vi "GlueRepeatedLinePattern.vi"(2 "Controller In":refnum<k24>, 3 "Dry Run":bool, 4 "Stereo Angle [mrad]":dbl=-26.0 format="%#_13g", 5 "Module Number":i32=7, 6 "Calibration Directory":path) -> (0 ".NET Refnum out":refnum<k24>)   [LabVIEW 2016]
uses:
  <vilib>/LabVIEW Interface for Arduino/Type Defs/Arduino Resource.ctl
  <vilib>/LabVIEW Interface for Arduino/Type Defs/Board Type.ctl
  C:/Users/Aerotech/Documents/BNLStaveAssembly-blueprint/Bin/Aerotech.A3200.dll
  BNLStaveAssembly-blueprint/Bin/Aerotech.A3200.dll
  <vilib>/LabVIEW Interface for Arduino/Type Defs/Pin Mode.ctl
  <vilib>/Utility/file.llb/Read Delimited Spreadsheet (DBL).vi
  <vilib>/LabVIEW Interface for Arduino/LabVIEW Interface for Arduino.lvlib
panel:
  out "Shift to Start [mm]":dbl[](array[numeric])
  out "Calibrated Start [mm]":dbl[](array[numeric])
  out "Start Position [mm]":dbl[](array[numeric])
  out "Line Motion":T1
  out "N Lines":i32
  out "Lines Glued":i32
  out "Elapsed Time [s]":dbl format="%.2g"
  out "Finished":bool
  in  "Abort stage":bool
  in  "Pattern Indicator":enum32{"Glue Pattern"}(tab)
  out "Relative Line\nSeparations [mm]":dbl[][](array[numeric])=[[18.5, 7.25], [2.5, 3.5], [-3.5, 5.0], [2.5, 3.15], [2.5, 3.15], [2.5, 3.15], [2.5, 3.15], [2.5, 3.15], [2.5, 3.15], [2.5, 3.15], [2.5, 3.15], [2.5, 3.15], [2.5, 3.15], [2.5, 3.15], [3.75, 5.0], [2.5, 3.5]] format="%#_13g"
  out "Line Lengths [mm]":dbl[](array[numeric])=[65.0, 65.0, 73.5, 73.5, 73.5, 73.5, 73.5, 73.5, 73.5, 73.5, 73.5, 73.5, 73.5, 73.5, 65.0, 65.0] format="%#_13g"
  in  "Outputs Tab":enum32{"Running Positions"}(tab)
  out "Running Positions [mm]":dbl[][](array[numeric])
  in  "Times [s]":dbl[](array[numeric])
  out "Running Times [s]":dbl[](array[numeric])
  in  "Inputs Tab":T2(tab)
  out "Virtual Stave Map":path
  out "Stave Angle [rad]":dbl format="%#_13g"
  out "Total Angle [rad]":dbl
  out "Orientation":string
  out "Pin Down?":bool
  in  "Pulse Length [ms]":dbl=125.0 format="%#_13g"
  out "Arduino Resource":T3={"VISA resource"="GlueCTRL", "Board Type"=enum."Uno", "Connection Type"=enum."USB / Serial", "Bytes Per Packet (15)"=15}
  in  "Digital I/O Pin":u8=7
  in  "Default Axis Speeds":T5={"X [mm/s]"=25.0, "Y [mm/s]"=25.0, "Z [mm/s]"=25.0}
  in  "Camera to Dispenser \nShift [mm]":dbl[](array[numeric])=[109.832, 5.121, 0.0]
  in  "Glue Pattern .csv File":path=path "C:/Users/Aerotech/Documents/BNL_ThermomechanicalStave/Glue/GluePatterns/Pattern6-0.txt"
  in  "Axial":bool=TRUE
  in  "Motion Time per Line [s]":dbl=4.35 format="%#_13g"
  in  "Wait [ms]":dbl=750.0 format="%#_13g"
  in  "Positions [mm]":dbl[][](array[numeric])
  in  "Terminate":bool
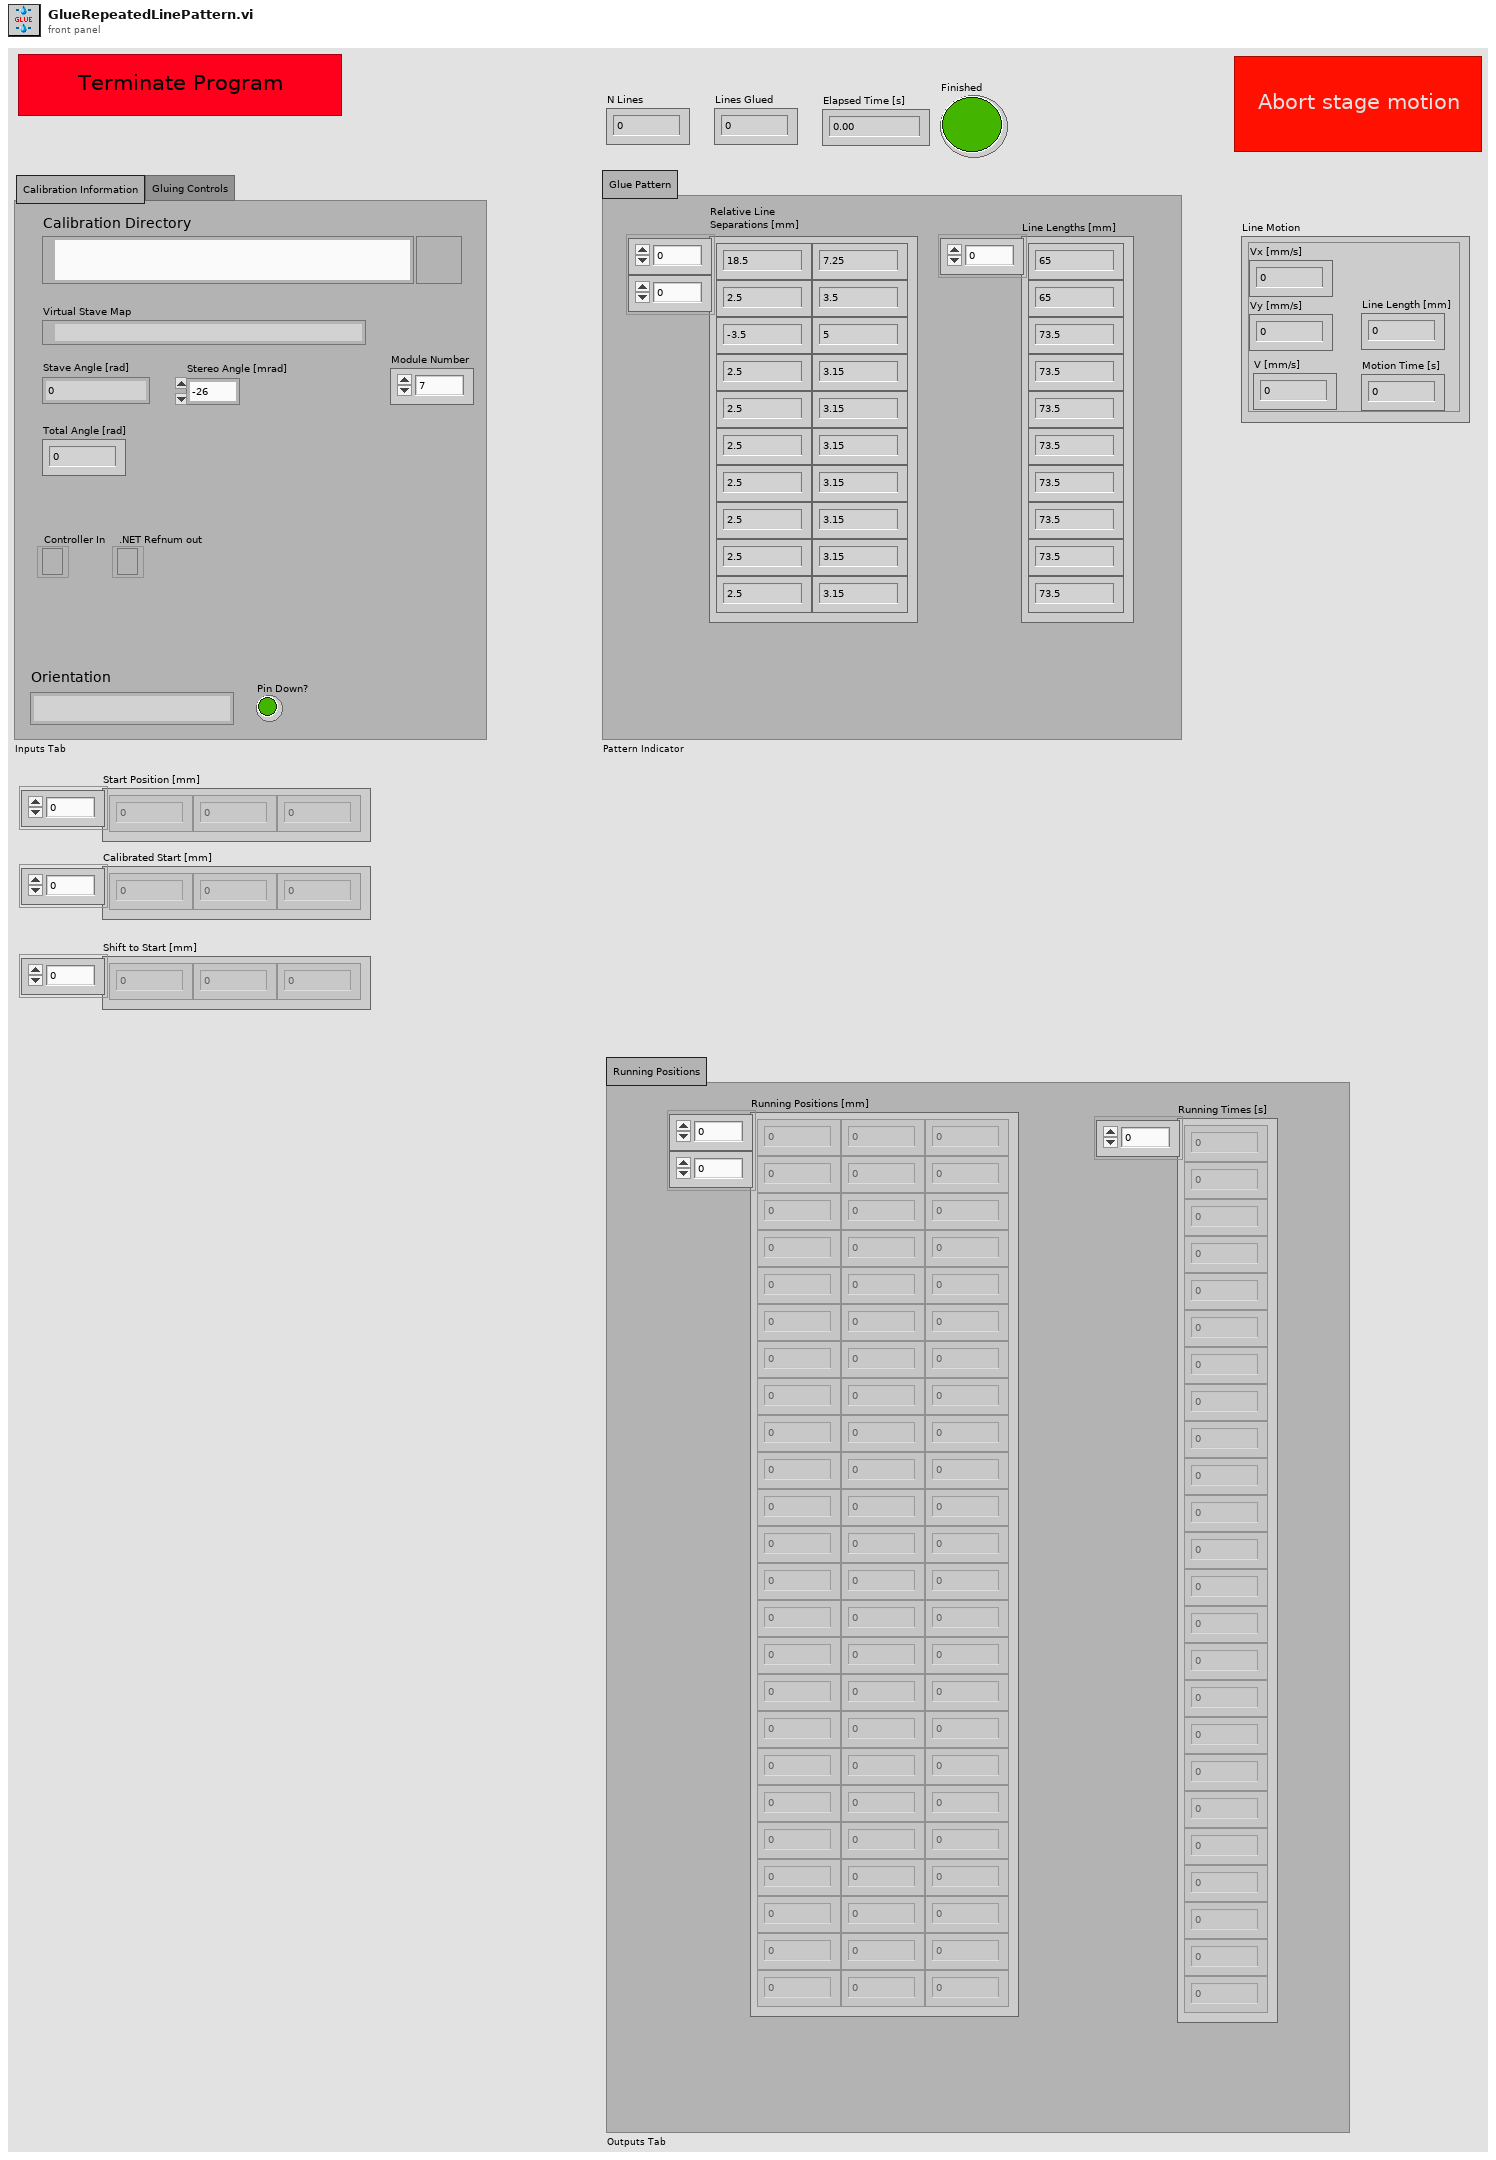
[diagram p1: front panel]
types:
  T1 = cluster{"Vx [mm/s]":dbl, "Vy [mm/s]":dbl, "Numeric Control":dbl, "Numeric Control":dbl, "Line Length [mm]":dbl}
  T2 = enum32{"Calibration Information", "Gluing Controls"}
  T3 = typedef "LabVIEW Interface for Arduino.lvlib/Arduino Resource.ctl" = cluster{"VISA resource":refnum<visa-resource-name>, "Board Type":T4, "Connection Type":enum8{"USB / Serial"}, "Bytes Per Packet (15)":u8}
  T4 = typedef "LabVIEW Interface for Arduino.lvlib/Board Type.ctl" = enum16{"Uno", "Dimuelanove w/Atmega 328", "Mega 2560"}
  T5 = cluster{"X [mm/s]":dbl, "Y [mm/s]":dbl, "Z [mm/s]":dbl}
  T6 = typedef "LabVIEW Interface for Arduino.lvlib/Pin Mode.ctl" = enum8{"Input", "Output"}
  T7 = cluster{"X [mm]":dbl, "Y [mm]":dbl, "Z [mm]":dbl}
  T8 = cluster{"Final X":dbl, "Final Y":dbl, "Final Z":dbl}
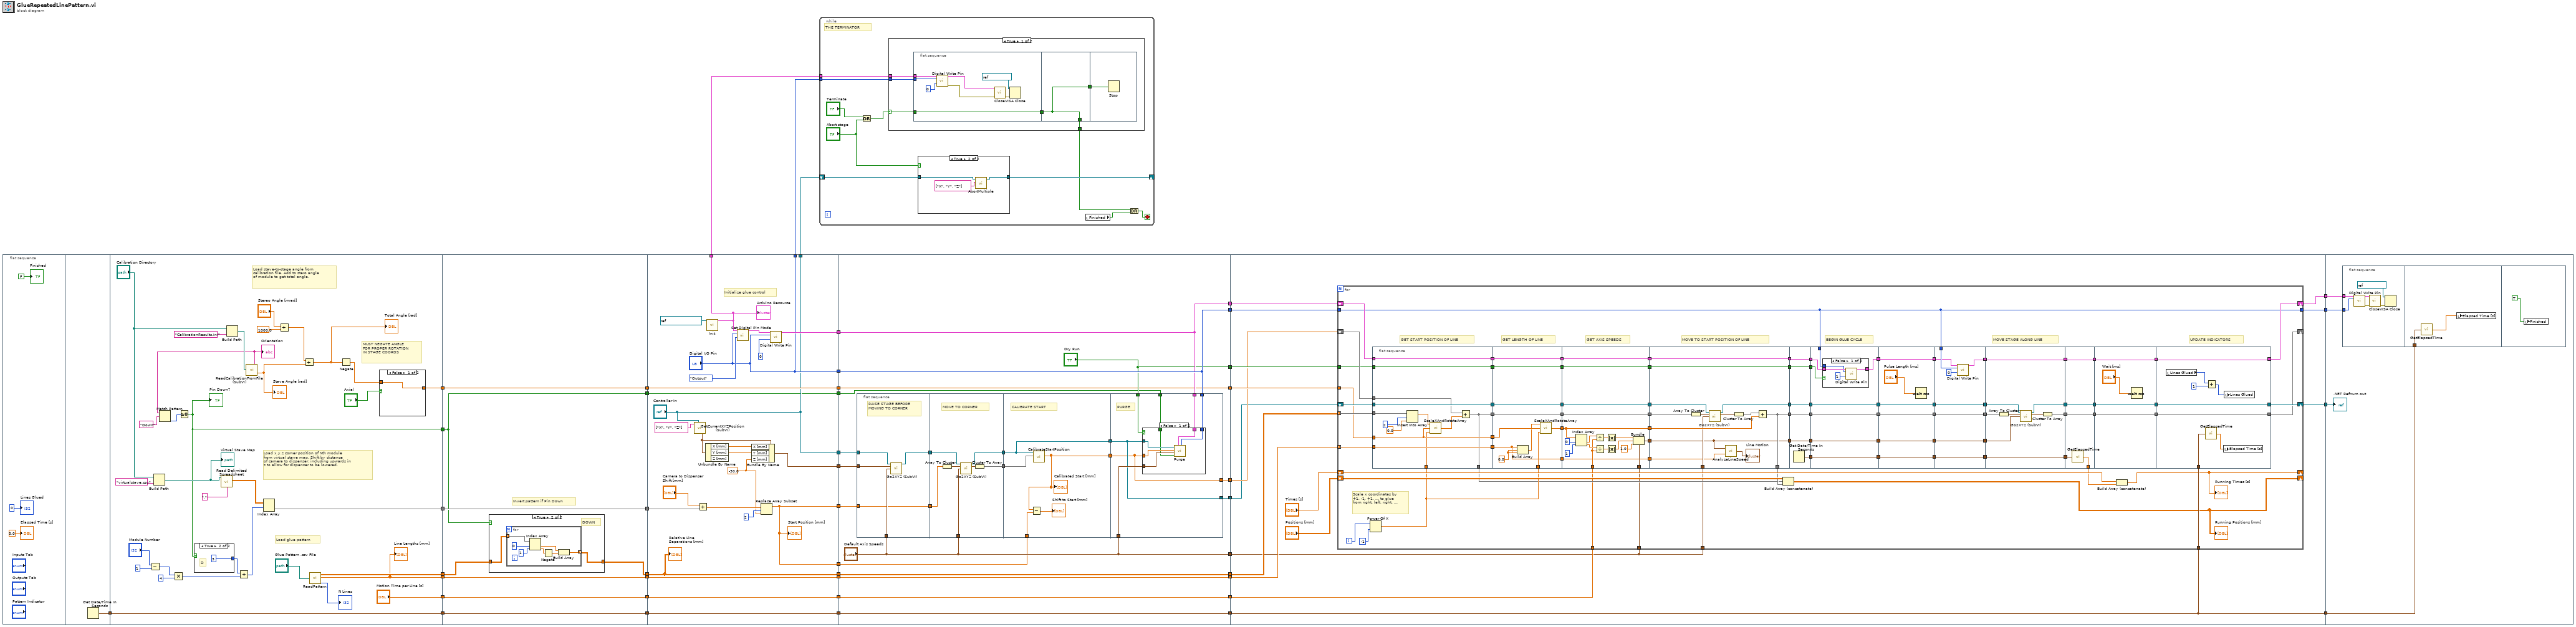
[diagram p0: block diagram]
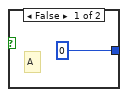
[diagram p2: hidden frame]
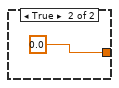
[diagram p3: hidden frame]
diagram:
  n1 = flat-sequence {
    tunnel: [w49] -> w31
    tunnel: w31 -> [w69]
    tunnel: [w69] -> w16
    tunnel: [w63] -> w14
    tunnel: [w66] -> w12
    tunnel: [w65] -> w10
    tunnel: [w62] -> w8
    tunnel: ["Motion Time per Line [s]"] -> w6
    tunnel: [w50] -> w4
    tunnel: w16 -> [w94]
    tunnel: [w94] -> w15
    tunnel: w14 -> [w93]
    tunnel: [w93] -> w13
    tunnel: w12 -> [w89]
    tunnel: [w88] -> w11
    tunnel: w10 -> [w92]
    tunnel: [w92] -> w9
    tunnel: w8 -> [w91]
    tunnel: [w91] -> w7
    tunnel: w6 -> [w90]
    tunnel: [w90] -> w5
    tunnel: w4 -> [w87]
    tunnel: [w87] -> w3
    tunnel: ["Controller In"] -> w45
    tunnel: [w125] -> w44
    tunnel: ["Digital I/O Pin"] -> w43
    tunnel: [w124] -> w37
    tunnel: ["Controller In"] -> w36
    tunnel: [w122] -> w33
    tunnel: w15 -> [w123]
    tunnel: [w123] -> w30
    tunnel: w13 -> [w122]
    tunnel: ["Digital I/O Pin"] -> w27
    tunnel: [w107] -> w24
    tunnel: w11 -> [w107]
    tunnel: w9 -> [w120]
    tunnel: [w120] -> w23
    tunnel: w7 -> [w113]
    tunnel: w5 -> [w119]
    tunnel: [w119] -> w22
    tunnel: [w105] -> w19
    tunnel: [w111] -> w18
    tunnel: w3 -> [w106]
    tunnel: [w106] -> w2
    tunnel: [w105] -> w1
    tunnel: w45 -> [w147]
    tunnel: w44 -> [w145]
    tunnel: w43 -> [w146]
    tunnel: [w146] -> w40
    tunnel: [w145] -> w39
    tunnel: [w144] -> w38
    tunnel: ["Dry Run"] -> w35
    tunnel: [w142] -> w34
    tunnel: w33 -> [w142]
    tunnel: [w141] -> w32
    tunnel: w30 -> [w140]
    tunnel: [w140] -> w29
    tunnel: [w139] -> w26
    tunnel: [w138] -> w25
    tunnel: w24 -> [w139]
    tunnel: w23 -> [w138]
    tunnel: w22 -> [w136]
    tunnel: [w136] -> w21
    tunnel: ["Default Axis Speeds"] -> w20
    tunnel: w19 -> [w133]
    tunnel: w18 -> [w132]
    tunnel: w2 -> [w131]
    tunnel: w1 -> [w130]
    tunnel: [w184] -> w42
    tunnel: [w196] -> w41
    tunnel: w40 -> [w195]
    tunnel: w39 -> [w194]
    tunnel: w38 -> [w190]
    tunnel: w35 -> [w193]
    tunnel: w34 -> [w192]
    tunnel: w32 -> [w191]
    tunnel: w29 -> [w189]
    tunnel: [w189] -> w28
    tunnel: w26 -> [w188]
    tunnel: w25 -> [w187]
    tunnel: w21 -> [w185]
    tunnel: w20 -> [w183]
    tunnel: [w182] -> w17
    tunnel: w42 -> [w395]
    tunnel: w41 -> [w394]
    tunnel: w28 -> [w393]
    tunnel: w17 -> [w392]
    frame #0 {
      "Finished" <- FALSE ("Finished")
      "Elapsed Time [s]" <- 0.0 ("Elapsed Time [s]")
      "Lines Glued" <- 0 ("N Lines")
    }
    frame #1 {
      n2 = Get Date/Time In Seconds() -> (seconds since 1Jan1904=w49:timestamp)
    }
    frame #2 {
      # "MUST NEGATE ANGLE \nFOR PROPER ROTATION\nIN STAGE COORDS"
      # "Load glue pattern"
      # "Load x,y,z corner position of Nth module\nfrom virtual stave map. Shift by distance\nof camera to dispenser, including upwards in\nz to allow for dispenser to be lowered."
      # "Load stave-to-stage angle from\ncalibration file. Add to stero angle\nof module to get total angle."
      n3 = Subtract(x="Module Number", y=1) -> (x-y=w72:i32)
      n4 = Build Path(base path="Calibration Directory", name or relative path="virtualstave.csv") -> (appended path=w76:path)
      "Virtual Stave Map" <- w76
      n5 = Multiply(x=w72, y=4) -> (x*y=w56:i32)
      n6 = call-poly <vilib>:"Read Delimited Spreadsheet.vi"("file path (dialog if empty)"=w76, "delimiter (\\t)"="," ("delimiter (\\t)")) -> ("all rows"=w70:dbl[][])  [unwired: 8 in, 5 out]
      n7 = Build Path(base path="Calibration Directory", name or relative path="CalibrationResults.ini") -> (appended path=w78:path)
      n8 = call "ReadCalibrationFromFile (SubVI).vi"("Calibration file path"=w78) -> ("Orientation"=w52:string, "Angle"=w60:dbl)  [unwired: 11 in, 6 out]
      "Stave Angle [rad]" <- w60
      "Orientation" <- w52
      n9 = Match Pattern(string=w52, regular expression="Down") -> (offset past match=w53:i32)  [unwired: 1 in, 3 out]
      n10 = Greater Or Equal To 0?(x=w53) -> (x >= 0?=w50:bool)
      "Pin Down?" <- w50
      n11 = case shown="True" w50 {
        tunnel: [0 3] -> w51
        frame False {
          # "A"
        }
        frame True {
          # "D"
        }
      }
      n12 = Add(x=w51, y=w56) -> (x+y=w55:i32)
      n13 = Index Array(array=w70, index (row)=w55) -> (element=w62:dbl[])  [unwired: 1 in]
      n14 = Divide(x="Stereo Angle [mrad]", y=1000.0) -> (x/y=w59:dbl)
      n15 = Add(x=w59, y=w60) -> (x+y=w58:dbl)
      "Total Angle [rad]" <- w58
      n16 = call "ReadPattern.vi"("file path (dialog if empty)"="Glue Pattern .csv File") -> ("Relative Line\nSeparations [mm]"=w66:dbl[][], "Line Lengths [mm]"=w65:dbl[], "N Lines"=→"N Lines":i32)  [unwired: 1 in]
      "Line Lengths [mm]" <- w65
      n17 = Negate(x=w58) -> (-x=w57:dbl)
      n18 = case shown="False" "Axial" {
        tunnel: [w85 0.0] -> w63
        tunnel: w57 -> [w85 _]
        frame False {
        }
        frame True {
        }
      }
    }
    frame #3 {
      # "Invert pattern if Pin Down"
      n19 = case shown="True" w87 {
        tunnel: w89 -> [w95 w97]
        tunnel: [w95 w96] -> w88
        frame False {
          # "UP"
        }
        frame True {
          # "DOWN"
          n20 = for {
            tunnel: w97 -> [w104] mode=indexing
            tunnel: [w98] -> w96 mode=indexing
            n21 = Index Array(array=w104, index #1=0 ("index"), index #2=1 ("index")) -> (element #1=w100:dbl, element #2=w101:dbl)
            n22 = Negate(x=w101) -> (-x=w99:dbl)
            n23 = Build Array(w100, w99) -> (w98:dbl[])
          }
        }
      }
    }
    frame #4 {
      w108 = -30.0 ("Z [mm]")
      # "Initialize glue control"
      n24 = call "GetCurrentXYZPosition (SubVI).vi"(".NET Refnum in - Device"="Controller In", "Axes Names"=string[] ["X", "Y", "Z"]) -> ("Current stage position"=w116:T7)  [unwired: 4 in, 5 out]
      n25 = Add(x="Camera to Dispenser \nShift [mm]", y=w113) -> (x+y=w110:dbl[])
      n26 = Unbundle By Name(w116) -> ("X [mm]"=w115:dbl, "Y [mm]"=w114:dbl)  [unwired: 1 out]
      n27 = call <vilib>:"Init.vi"("VISA resource"=refnum<visa-resource-name> "GlueCTRL") -> ("Arduino Resource"=w124:T3)  [unwired: 17 in, 1 out]
      "Arduino Resource" <- w124
      n28 = call <vilib>:"Set Digital Pin Mode.vi"("Arduino Resource"=w124, "Digital I/O Pin"="Digital I/O Pin", "Pin Mode (Input)"=Pin_Mode."Output") -> ("Arduino Resource"=w127:T3)  [unwired: 11 in, 1 out]
      n29 = Bundle By Name(cluster=w116, "X [mm]"=w115, "Y [mm]"=w114, "Z [mm]"=w108) -> (w111:T7)
      n30 = Replace Array Subset(array=w110, new element=w108, index=2) -> (w105:dbl[])
      "Start Position [mm]" <- w105
      n31 = call <vilib>:"Digital Write Pin.vi"("Arduino Resource"=w127, "Digital I/O Pin (0)"="Digital I/O Pin", "Value (0)"=u8 0) -> ("Arduino Resource"=w125:T3)  [unwired: 11 in, 1 out]
      "Relative Line\nSeparations [mm]" <- w107
    }
    frame #5 {
      n32 = flat-sequence {
        tunnel: w147 -> [w156]
        tunnel: [w155] -> w137
        tunnel: "Default Axis Speeds" -> [w154]
        tunnel: [w153] -> w134
        tunnel: w133 -> [w153]
        tunnel: w132 -> [w152]
        tunnel: [w160] -> w151
        tunnel: [w159] -> w150
        tunnel: w137 -> [w161]
        tunnel: "Default Axis Speeds" -> [w158]
        tunnel: w134 -> [w157]
        tunnel: w151 -> [w167]
        tunnel: w150 -> [w168]
        tunnel: [w167] -> w149
        tunnel: [w166] -> w148
        tunnel: w130 -> [w165]
        tunnel: w149 -> [w172]
        tunnel: w148 -> [w170]
        tunnel: "Default Axis Speeds" -> [w175]
        tunnel: w146 -> [w174]
        tunnel: w145 -> [w173]
        tunnel: [w172] -> w144
        tunnel: "Dry Run" -> [w171]
        tunnel: [w170] -> w141
        tunnel: w131 -> [w169]
        frame #0 {
          # "RAISE STAGE BEFORE\nMOVING TO CORNER"
          n33 = call "Go2XYZ (SubVI).vi"(".NET Refnum in"=w156, "Go to Coordinates"=w152, "Axis Speeds"=w154) -> (".NET Refnum out"=w155:refnum<k24>)  [unwired: 8 in, 4 out]
        }
        frame #1 {
          # "MOVE TO CORNER"
          n34 = Array To Cluster(array=w157) -> (cluster=w163:cluster{"[0]":dbl, "[1]":dbl, "[2]":dbl})
          n35 = call "Go2XYZ (SubVI).vi"(".NET Refnum in"=w161, "Go to Coordinates"=w163, "Axis Speeds"=w158) -> (".NET Refnum out"=w160:refnum<k24>, "Final Position"=w162:T8)  [unwired: 8 in, 3 out]
          n36 = Cluster To Array(cluster=w162) -> (array=w159:dbl[])
        }
        frame #2 {
          # "CALIBRATE START"
          n37 = call "CalibrateStartPosition.vi"("Start Position [mm]"=w168, ".NET Refnum In"=w167) -> ("Final Position [mm]"=w166:dbl[])  [unwired: 9 in]
          "Calibrated Start [mm]" <- w166
          n38 = Subtract(x=w166, y=w165) -> (x-y=→"Shift to Start [mm]":dbl[])
        }
        frame #3 {
          # "PURGE"
          n39 = case shown="False" w171 {
            tunnel: w175 -> [w179 _]
            tunnel: w174 -> [w181 _]
            tunnel: w173 -> [w180 _]
            tunnel: w172 -> [w177 _]
            tunnel: w170 -> [w178 _]
            tunnel: w169 -> [w176 _]
            frame False {
              n40 = call "Purge.vi"("Digital I/O Pin"=w181, "Arduino Resource"=w180, "Pin Down?"=w176, "Axis Speeds"=w179, "Start Position [mm]"=w178, ".NET Refnum In"=w177) -> ()  [unwired: 6 in]
            }
            frame True {
            }
          }
        }
      }
    }
    frame #6 {
      n41 = for {
        tunnel: w188 -> [w233] mode=indexing
        tunnel: w187 -> [w231] mode=indexing
        shift-right: [w271] -> _
        shift-left: w191 -> [w234]
        shift-right: [w272] -> w182
        shift-left: w190 -> [w275]
        shift-right: [w276] -> w184
        shift-left: w194 -> [w274]
        shift-right: [w252] -> _
        shift-left: "Positions [mm]" -> [w273]
        tunnel: w195 -> [w251]
        tunnel: [w251] -> w196
        tunnel: w193 -> [w230]
        tunnel: w192 -> [w229]
        tunnel: w189 -> [w269]
        shift-right: [w253] -> _
        shift-left: "Times [s]" -> [w264]
        tunnel: w185 -> [w208]
        tunnel: w183 -> [w201]
        tunnel: w183 -> [w200]
        i -> [w270]
        # "GET AXIS SPEEDS"
        # "BEGIN GLUE CYCLE"
        # "GET LENGTH OF LINE"
        # "GET START POSITION OF LINE"
        # "UPDATE INDICATORS"
        # "MOVE STAGE ALONG LINE"
        # "MOVE TO START POSITION OF LINE"
        # "Scale x coordinates by\n+1, -1, +1, ... to glue\nfrom right, left, right, ..."
        n42 = Power Of X(1:-1 ("x"), 2:w270) -> (0:w227:dbl)
        n43 = flat-sequence {
          tunnel: w230 -> [w288]
          tunnel: w275 -> [w289]
          tunnel: w274 -> [w290]
          tunnel: [w290] -> w238
          tunnel: [w289] -> w237
          tunnel: [w288] -> w236
          tunnel: [w278] -> w235
          tunnel: w234 -> [w287]
          tunnel: w233 -> [w284]
          tunnel: [w281] -> w232
          tunnel: w231 -> [w281]
          tunnel: w229 -> [w280]
          tunnel: [w280] -> w228
          tunnel: w227 -> [w279]
          tunnel: [w278] -> w225
          tunnel: [w300] -> w224
          tunnel: [w299] -> w222
          tunnel: [w298] -> w220
          tunnel: [w297] -> w218
          tunnel: [w296] -> w216
          tunnel: w238 -> [w300]
          tunnel: w237 -> [w299]
          tunnel: w236 -> [w298]
          tunnel: w235 -> [w297]
          tunnel: w232 -> [w291]
          tunnel: w228 -> [w294]
          tunnel: w227 -> [w292]
          tunnel: [w291] -> w198
          tunnel: w224 -> [w318]
          tunnel: [w318] -> w223
          tunnel: w222 -> [w317]
          tunnel: [w317] -> w221
          tunnel: w220 -> [w316]
          tunnel: [w316] -> w219
          tunnel: w218 -> [w315]
          tunnel: [w315] -> w217
          tunnel: w216 -> [w313]
          tunnel: [w313] -> w215
          tunnel: w208 -> [w308]
          tunnel: [w307] -> w207
          tunnel: w200 -> [w302]
          tunnel: [w301] -> w199
          tunnel: w198 -> [w301]
          tunnel: [w332] -> w268
          tunnel: [w323] -> w267
          tunnel: [w326] -> w266
          tunnel: [w331] -> w265
          tunnel: w223 -> [w332]
          tunnel: w221 -> [w324]
          tunnel: w219 -> [w331]
          tunnel: w217 -> [w325]
          tunnel: w215 -> [w327]
          tunnel: [w326] -> w226
          tunnel: w207 -> [w319]
          tunnel: [w319] -> w204
          tunnel: w201 -> [w322]
          tunnel: w199 -> [w321]
          tunnel: w268 -> [w338]
          tunnel: [w338] -> w262
          tunnel: w267 -> [w337]
          tunnel: [w337] -> w261
          tunnel: w266 -> [w336]
          tunnel: [w336] -> w260
          tunnel: w265 -> [w335]
          tunnel: [w335] -> w259
          tunnel: [w334] -> w258
          tunnel: [w333] -> w205
          tunnel: w204 -> [w333]
          tunnel: w262 -> [w343]
          tunnel: w261 -> [w346]
          tunnel: [w346] -> w246
          tunnel: w260 -> [w345]
          tunnel: [w345] -> w244
          tunnel: w259 -> [w341]
          tunnel: w258 -> [w344]
          tunnel: [w344] -> w242
          tunnel: w251 -> [w340]
          tunnel: [w342] -> w240
          tunnel: [w339] -> w206
          tunnel: w205 -> [w339]
          tunnel: w246 -> [w357]
          tunnel: [w357] -> w245
          tunnel: w244 -> [w356]
          tunnel: [w356] -> w243
          tunnel: w242 -> [w355]
          tunnel: [w355] -> w241
          tunnel: w240 -> [w354]
          tunnel: [w354] -> w239
          tunnel: w206 -> [w352]
          tunnel: [w352] -> w202
          tunnel: w245 -> [w365]
          tunnel: [w365] -> w257
          tunnel: w243 -> [w364]
          tunnel: [w364] -> w256
          tunnel: w241 -> [w363]
          tunnel: [w363] -> w255
          tunnel: w239 -> [w360]
          tunnel: [w359] -> w254
          tunnel: w251 -> [w361]
          tunnel: [w358] -> w203
          tunnel: w202 -> [w358]
          tunnel: [w366] -> w250
          tunnel: w257 -> [w367]
          tunnel: w256 -> [w374]
          tunnel: [w373] -> w249
          tunnel: [w372] -> w248
          tunnel: w255 -> [w372]
          tunnel: w254 -> [w371]
          tunnel: [w371] -> w247
          tunnel: w203 -> [w370]
          tunnel: [w375] -> w214
          tunnel: w250 -> [w379]
          tunnel: [w379] -> w212
          tunnel: w249 -> [w378]
          tunnel: [w378] -> w210
          tunnel: w248 -> [w377]
          tunnel: [w376] -> w263
          tunnel: w247 -> [w375]
          tunnel: w214 -> [w383]
          tunnel: [w383] -> w213
          tunnel: w212 -> [w382]
          tunnel: [w382] -> w211
          tunnel: w210 -> [w381]
          tunnel: [w381] -> w209
          tunnel: [w391] -> w276
          tunnel: w213 -> [w391]
          tunnel: [w390] -> w272
          tunnel: w211 -> [w390]
          tunnel: [w389] -> w271
          tunnel: w209 -> [w389]
          tunnel: w269 -> [w385]
          frame #0 {
            n44 = Insert Into Array(array=w284, index=2, new element=0.0 ("new element/subarray")) -> (w283:dbl[])
            n45 = call "ScaleXAndRotateArray.vi"("Scale"=w279, "Angle"=w280, "X, Y, Z Input"=w283) -> ("c * X', Y', Z Output"=w282:dbl[])
            n46 = Add(x=w287, y=w282) -> (x+y=w278:dbl[])
          }
          frame #1 {
            w295 = 0.0 ("element")
            n47 = Build Array(w291, w295, w295) -> (w293:dbl[])
            n48 = call "ScaleXAndRotateArray.vi"("Scale"=w292, "Angle"=w294, "X, Y, Z Input"=w293) -> ("c * X', Y', Z Output"=w296:dbl[])
          }
          frame #2 {
            n49 = Index Array(array=w313, index #1=0 ("index"), index #2=1 ("index")) -> (element #1=w310:dbl, element #2=w309:dbl)
            n50 = Divide(x=w310, y=w308) -> (x/y=w306:dbl)
            n51 = Divide(x=w309, y=w308) -> (x/y=w305:dbl)
            n52 = Absolute Value(x=w306) -> (abs(x)=w304:dbl)
            n53 = Absolute Value(x=w305) -> (abs(x)=w303:dbl)
            n54 = Bundle(cluster=w302, "X [mm/s]"=w304, "Y [mm/s]"=w303, "Z [mm/s]"=1.0) -> (w307:T5)
          }
          frame #3 {
            n55 = Array To Cluster(array=w325) -> (cluster=w328:cluster{"[0]":dbl, "[1]":dbl, "[2]":dbl})
            n56 = call "Go2XYZ (SubVI).vi"(".NET Refnum in"=w324, "Go to Coordinates"=w328, "Axis Speeds"=w322) -> (".NET Refnum out"=w323:refnum<k24>, "Final Position"=w329:T8)  [unwired: 8 in, 3 out]
            n57 = call "AnalyzeLineSpeed.vi"("Line Length [mm]"=w321, "Line Speeds [mm/s]"=w319) -> ("Output"=→"Line Motion":T1)
            n58 = Cluster To Array(cluster=w329) -> (array=w330:dbl[])
            n59 = Add(x=w330, y=w327) -> (x+y=w326:dbl[])
          }
          frame #4 {
            n60 = Get Date/Time In Seconds() -> (seconds since 1Jan1904=w334:timestamp)
          }
          frame #5 {
            n61 = case shown="False" w341 {
              tunnel: [w350 w351] -> w342
              tunnel: w343 -> [w349 w351]
              tunnel: w340 -> [w347 _]
              frame False {
                n62 = call <vilib>:"Digital Write Pin.vi"("Arduino Resource"=w349, "Digital I/O Pin (0)"=w347, "Value (0)"=u8 1) -> ("Arduino Resource"=w350:T3)  [unwired: 11 in, 1 out]
              }
              frame True {
              }
            }
          }
          frame #6 {
            n63 = Wait (ms)(milliseconds to wait="Pulse Length [ms]") -> ()  [unwired: 1 out]
          }
          frame #7 {
            n64 = call <vilib>:"Digital Write Pin.vi"("Arduino Resource"=w360, "Digital I/O Pin (0)"=w361, "Value (0)"=u8 0) -> ("Arduino Resource"=w359:T3)  [unwired: 11 in, 1 out]
          }
          frame #8 {
            n65 = Array To Cluster(array=w374) -> (cluster=w368:cluster{"[0]":dbl, "[1]":dbl, "[2]":dbl})
            n66 = call "Go2XYZ (SubVI).vi"(".NET Refnum in"=w367, "Go to Coordinates"=w368, "Axis Speeds"=w370) -> (".NET Refnum out"=w366:refnum<k24>, "Final Position"=w369:T8)  [unwired: 8 in, 3 out]
            n67 = Cluster To Array(cluster=w369) -> (array=w373:dbl[])
          }
          frame #9 {
            n68 = call "GetElapsedTime.vi"("Start Time"=w377) -> ("Elapsed Time [s]"=w376:sgl)
          }
          frame #10 {
            n69 = Wait (ms)(milliseconds to wait="Wait [ms]") -> ()  [unwired: 1 out]
          }
          frame #11 {
            n70 = local read "Lines Glued"() -> (w387:i32)
            n71 = call "GetElapsedTime.vi"("Start Time"=w385) -> ("Elapsed Time [s]"=w384:sgl)
            n72 = Add(x=w387, y=1) -> (x+y=w388:i32)
            n73 = local write "Elapsed Time [s]"(w384) -> ()
            n74 = local write "Lines Glued"(w388) -> ()
          }
        }
        n75 = Build Array (concatenate)(w273, w225, w226) -> (w252:dbl[][])
        "Running Positions [mm]" <- w252
        n76 = Build Array (concatenate)(w264, w263) -> (w253:dbl[])
        "Running Times [s]" <- w253
      }
    }
    frame #7 {
      n77 = flat-sequence {
        tunnel: w395 -> [w397]
        tunnel: w394 -> [w396]
        tunnel: w393 -> [w402]
        frame #0 {
          n78 = call <vilib>:"Digital Write Pin.vi"("Arduino Resource"=w397, "Digital I/O Pin (0)"=w396) -> ("Arduino Resource"=w400:T3, "error out"=w399:errorcluster)  [unwired: 12 in]
          n79 = call <vilib>:"Close.vi"("Arduino Resource"=w400, "error in"=w399) -> ("error out"=w398:errorcluster)  [unwired: 13 in]
          n80 = VISA Close(VISA resource name=refnum<visa-resource-name> "GlueCTRL", error in (no error)=w398) -> ()  [unwired: 1 out]
        }
        frame #1 {
          n81 = call "GetElapsedTime.vi"("Start Time"=w402) -> ("Elapsed Time [s]"=w403:sgl)
          n82 = local write "Elapsed Time [s]"(w403) -> ()
        }
        frame #2 {
          n83 = local write "Finished"(TRUE ("stop? (T)")) -> ()
        }
      }
      ".NET Refnum out" <- w392
    }
  }
  n84 = while {
    tunnel: w37 -> [w414]
    shift-right: [w412] -> _
    shift-left: w36 -> [w413]
    tunnel: w27 -> [w406]
    stop <- w409 stop-if-true
    # "THE TERMINATOR"
    n85 = Or(x="Terminate", y="Abort stage") -> (x .or. y?=w408:bool)
    n86 = case shown="True" w408 {
      selector: w408 -> [w424 w435]
      tunnel: w414 -> [w422 _]
      tunnel: [w420 w435] -> w407
      tunnel: w406 -> [w419 _]
      frame True {
        n87 = flat-sequence {
          tunnel: [w430] -> w423
          tunnel: w419 -> [w426]
          tunnel: w422 -> [w428]
          tunnel: w424 -> [w430]
          tunnel: w423 -> [w433]
          tunnel: [w433] -> w421
          tunnel: [w433] -> w420
          tunnel: w421 -> [w434]
          frame #0 {
            n88 = call <vilib>:"Digital Write Pin.vi"("Arduino Resource"=w428, "Digital I/O Pin (0)"=w426, "Value (0)"=u8 0) -> ("Arduino Resource"=w429:T3, "error out"=w425:errorcluster)  [unwired: 11 in]
            n89 = call <vilib>:"Close.vi"("Arduino Resource"=w429, "error in"=w425) -> ("error out"=w431:errorcluster)  [unwired: 13 in]
            n90 = VISA Close(VISA resource name=refnum<visa-resource-name> "GlueCTRL", error in (no error)=w431) -> ()  [unwired: 1 out]
          }
          frame #1 {
          }
          frame #2 {
            n91 = Stop(stop? (T)=w434) -> ()
          }
        }
      }
      frame False {
      }
    }
    n92 = case shown="True" "Abort stage" {
      tunnel: w413 -> [w415 w417]
      tunnel: [w415 w416] -> w412
      frame False {
      }
      frame True {
        n93 = call "AbortMultiple.vi"("axis names"=string[] ["X", "Y", "Z"], "controller in"=w417) -> ("controller out"=w416:refnum<k24>)  [unwired: 8 in, 1 out]
      }
    }
    n94 = local read "Finished"() -> (w405:bool)
    n95 = Or(x=w407, y=w405) -> (x .or. y?=w409:bool)
  }
